vi "configuration_extended_depth.vi"() -> (3 "configuration_extended_depth":T1={"chunk"=4096, "media_index"=4294967295, "stride_mask"=63, "mode"=1, "divisor"=1, "profile_z"=1, "_reserved_0"=0, "_reserved_1"=0, "_reserved_2"=0, "_reserved_3"=0, "_reserved_4"=0})   [LabVIEW 2023]
panel:
  in  "configuration_extended_depth":T1={"chunk"=4096, "media_index"=4294967295, "stride_mask"=63, "mode"=1, "divisor"=1, "profile_z"=1, "_reserved_0"=0, "_reserved_1"=0, "_reserved_2"=0, "_reserved_3"=0, "_reserved_4"=0}
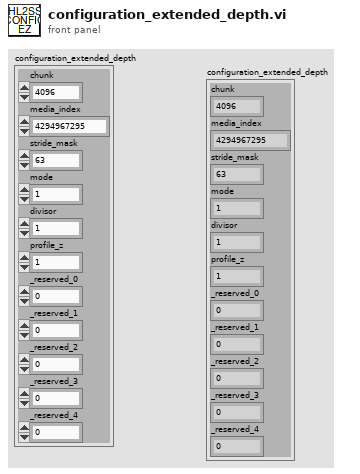
[diagram p1: front panel]
types:
  T1 = cluster{"chunk":u64, "media_index":u64, "stride_mask":u64, "mode":u8, "divisor":u8, "profile_z":u8, "_reserved_0":u8, "_reserved_1":u8, "_reserved_2":u8, "_reserved_3":u8, "_reserved_4":u8}
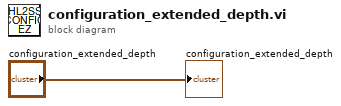
[diagram p0: block diagram]
diagram:
  "configuration_extended_depth" <- "configuration_extended_depth"
